vi "Dispatcher Read and Process UDP Messages.vi"(0 "UDP conn ID":refnum<k16>, 9 "timeout (10 ms)":i32=10, 11 "error in":errorcluster) -> (4 "message string":string, 6 "message":T1, 15 "error out":errorcluster)   [LabVIEW 2014, in "AMC.lvlib"]
uses:
  AMC.lvlib
  Message.ctl
  <vilib>/NI/Tools/Keyed Array/KeyedArray.ctl
  <vilib>/NI/Tools/Keyed Array/Tools_KeyedArray.lvlib
panel:
  out "message length":i32
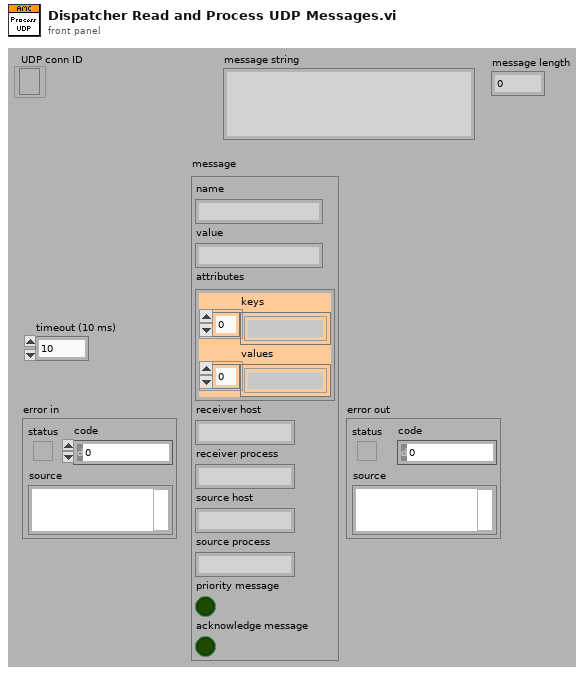
[diagram p1: front panel]
types:
  T1 = typedef "AMC.lvlib/Message.ctl" = cluster{"name":string, "value":string, "attributes":T2, "receiver host":string, "receiver process":string, "source host":string, "source process":string, "priority message":bool, "acknowledge message":bool}
  T2 = typedef "Tools_KeyedArray.lvlib/KeyedArray.ctl" = cluster{"keys":string[], "values":string[]}
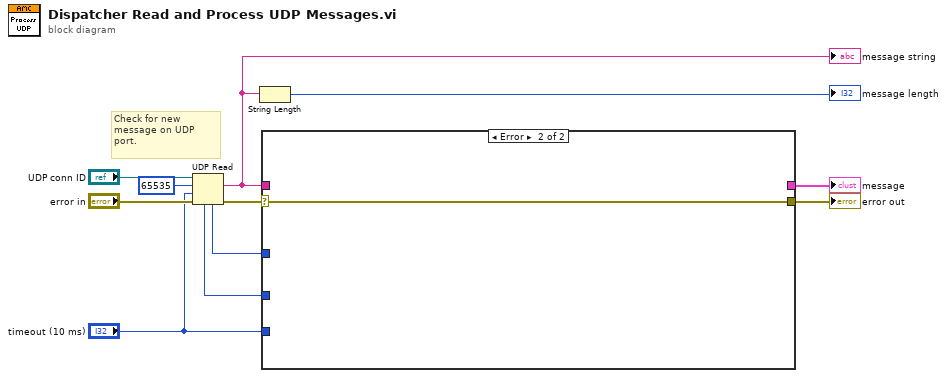
[diagram p0: block diagram]
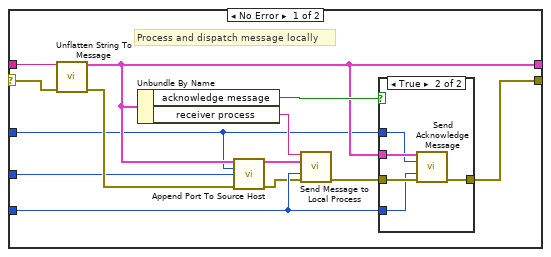
[diagram p2: hidden frame]
diagram:
  # "Check for new message on UDP port."
  n1 = UDP Read(connection ID="UDP conn ID", max size (548)=65535, timeout ms (25000)="timeout (10 ms)", 8:"error in") -> (data out=w4:string, error out=w10:errorcluster, 4:w2:u16, 6:w1:u32)  [unwired: 1 out]
  "message string" <- w4
  n2 = String Length(string=w4) -> (length=→"message length":i32)
  n3 = case shown="Error" w10 {
    selector: w10 -> [w23 w31]
    tunnel: w4 -> [w24 _]
    tunnel: [w20 w31] -> w8
    tunnel: [w17 _] -> w6
    tunnel: "timeout (10 ms)" -> [w18 _]
    tunnel: w2 -> [w13 _]
    tunnel: w1 -> [w12 _]
    frame No Error {
      # "Process and dispatch message locally"
      n4 = call "Unflatten String To Message.vi"("message string"=w24, "error in"=w23) -> ("message"=w17:T1, "error out"=w15:errorcluster)  [unwired: 12 in]
      n5 = Unbundle By Name(w17) -> ("acknowledge message"=w19:bool, "receiver process"=w22:string)
      n6 = call "Append Port To Source Host.vi"("message in"=w17, "source port"=w13, "source address"=w12, "error in"=w15) -> ("message out"=w16:T1, "error out"=w14:errorcluster)  [unwired: 10 in]
      n7 = call "Send Message to Local Process.vi"("process name"=w22, "message"=w16, "timeout (-1 ms)"=w18, "error in"=w14) -> ("error out"=w21:errorcluster)  [unwired: 10 in, 1 out]
      n8 = case shown="True" w19 {
        tunnel: w21 -> [w25 w30]
        tunnel: [w25 w29] -> w20
        tunnel: w17 -> [_ w28]
        tunnel: w13 -> [_ w27]
        tunnel: w18 -> [_ w26]
        frame False {
        }
        frame True {
          n9 = call "Send Acknowledge Message.vi"("received message"=w28, "receiver port"=w27, "timeout"=w26, "error in"=w30) -> ("error out"=w29:errorcluster)  [unwired: 10 in, 1 out]
        }
      }
    }
    frame Error {
    }
  }
  "error out" <- w8
  "message" <- w6
